vi "Begin.vi"(8 "error in":errorcluster) -> (0 "error out":errorcluster)   [LabVIEW 2016]
doc: "Called before other user functions, this VI is expected to open initial I/O refnums, load in file data, and do all program initialization. Notice that the <B>error out</B> terminal is simply used for data flow. Wiring it to other structures or subVIs ensures that this VI runs first."
uses:
  Robot Global Data.vi
  <vilib>/Rock Robotics/WPI/DriverStation/WPI_DriverStationRobotMode2.ctl
  <vilib>/Rock Robotics/WPI/Joystick/WPI_JoystickDeviceEnum.ctl
  <vilib>/Rock Robotics/Network Tables/NT Write String Array.vi
  <vilib>/Rock Robotics/WPI/SafetyOutput/WPI_SafetyOutputConfigMenu.ctl
  <vilib>/Rock Robotics/WPI/Solenoid/WPI_SolenoidOpenDouble.vi
  <vilib>/Rock Robotics/WPI/RobotDrive/WPI_RobotDriveOpen4MotorWithExistingMotors.vi
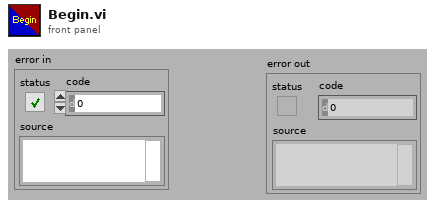
[diagram p1: front panel]
types:
  T1 = typedef "WPI_JoystickDeviceEnum.ctl" = enum16{"USB 0", "USB 1", "USB 2", "USB 3", "USB 4", "USB 5"}
  T2 = typedef "WPI_SafetyOutputConfigMenu.ctl" = enum16{"Enable", "Disable"}
  T3 = typedef "WPI_DriverStationRobotMode2.ctl" = enum16{"Autonomous Disabled", "Autonomous Enabled", "Teleop Disabled", "Teleop Enabled", "Disconnected", "Finish", "Test Disabled", "Test Enabled", "Emergency Stopped"}
  T4 = typedef "WPI_MotorControlDeviceRef.ctl" = cluster{"DeviceStatus":errorcluster, "Type":T5, "PWM":cluster{"PWM Channel":T6, "DeadBand":T7}, "CAN":cluster{"Device Number":u8, "SetOutput VI Ref":variant, "GetOutput VI Ref":variant, "Enable VI Ref":variant, "Disable VI Ref":variant, "Data":variant}, "Invert":bool}
  T5 = typedef "WPI_MotorControlType.ctl" = enum16{"PWM", "CAN"}
  T6 = typedef "FPGA_DIOPWMChannel.ctl" = enum8{"PWM 0", "PWM 1", "PWM 2", "PWM 3", "PWM 4", "PWM 5", "PWM 6", "PWM 7", "PWM 8", "PWM 9", "PWM MXP 0", "PWM MXP 1", "PWM MXP 2", "PWM MXP 3", "PWM MXP 4", "PWM MXP 5", "PWM MXP 6", "PWM MXP 7", "PWM MXP 8", "PWM MXP 9", "Invalid"}
  T7 = typedef "WPI_PWMDeadband.ctl" = cluster{"Name":string, "maxPositivePwm":i32, "minPositivePwm":i32, "centerPwm":i32, "maxNegativePwm":i32, "minNegativePwm":i32, "angularRange":u16}
  T8 = typedef "WPI_JoystickDevRef.ctl" = cluster{"Device":T1}
  T9 = typedef "WPI_RobotDriveDevRef.ctl" = cluster{"DevStatus":errorcluster, "Motors[]":T4[], "Square Inputs":bool, "Max Output":dbl}
  T10 = typedef "WPI_SolenoidDevRef.ctl" = cluster{"DevStatus":errorcluster, "Pneumatics Control Module":u8, "Forward Solenoid Channel":T11, "Reverse Solenoid Channel":T11}
  T11 = typedef "WPI_SolenoidChannel.ctl" = enum8{"Solenoid 0", "Solenoid 1", "Solenoid 2", "Solenoid 3", "Solenoid 4", "Solenoid 5", "Solenoid 6", "Solenoid 7", "Invalid"}
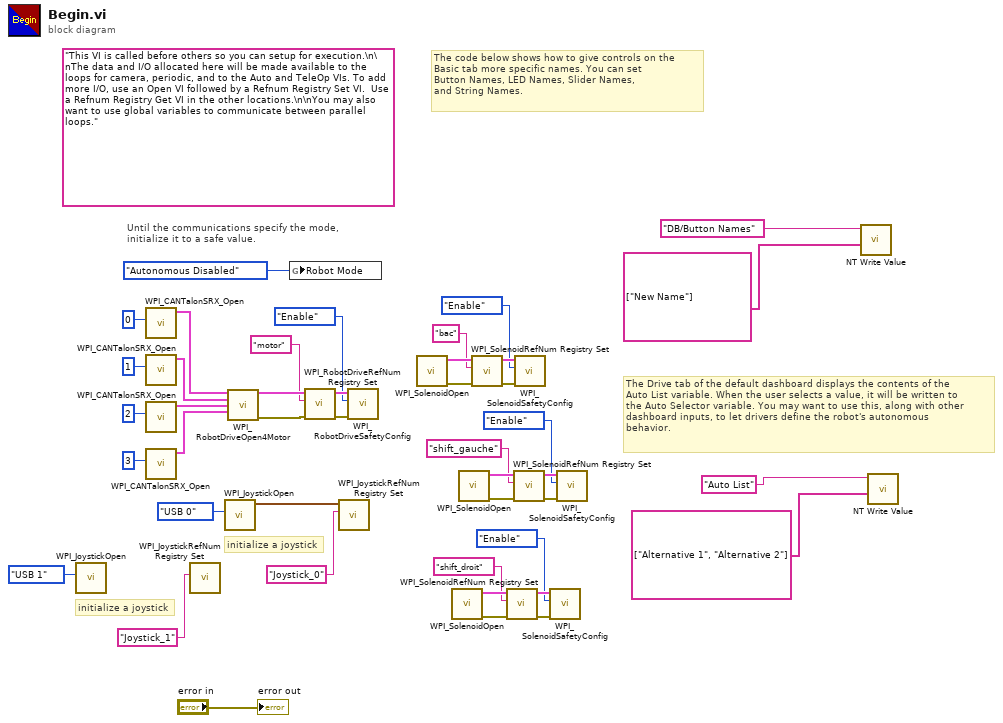
[diagram p0: block diagram]
diagram:
  (unwired) "This VI is called before others so you can setup for execution.\n\nThe data and I/O allocated here will be made available to the loops for camera, periodic, and to the Auto and TeleOp VIs. To add more I/O, use an Open VI followed by a Refnum Registry Set VI.  Use a Refnum Registry Get VI in the other locations.\n\nYou may also want to use global variables to communicate between parallel loops."
  # "initialize a joystick"
  # "The Drive tab of the default dashboard displays the contents of the\nAuto List variable. When the user selects a value, it will be written to\nthe Auto Selector variable. You may want to use this, along with other\ndashboard inputs, to let drivers define the robot's autonomous\nbehavior."
  # "The code below shows how to give controls on the\nBasic tab more specific names. You can set\nButton Names, LED Names, Slider Names,\nand String Names."
  # "initialize a joystick"
  # "Until the communications specify the mode,\ninitialize it to a safe value."
  n1 = call <vilib>:"WPI_JoystickOpen.vi"("JoystickDevice"=WPI_JoystickDeviceEnum."USB 1") -> ()  [unwired: 10 in, 1 out]
  n2 = call <vilib>:"WPI_CANTalonSRX_Open.vi"("Device Number"=u8 0) -> ("CAN Talon SRX Ref"=w29:T4)  [unwired: 9 in, 1 out]
  n3 = call <vilib>:"WPI_CANTalonSRX_Open.vi"("Device Number"=u8 1) -> ("CAN Talon SRX Ref"=w28:T4)  [unwired: 9 in, 1 out]
  n4 = call <vilib>:"WPI_CANTalonSRX_Open.vi"("Device Number"=u8 2) -> ("CAN Talon SRX Ref"=w27:T4)  [unwired: 9 in, 1 out]
  n5 = call <vilib>:"WPI_CANTalonSRX_Open.vi"("Device Number"=u8 3) -> ("CAN Talon SRX Ref"=w26:T4)  [unwired: 9 in, 1 out]
  n6 = call <vilib>:"WPI_JoystickRefNum Registry Set.vi"("refnum name"="Joystick_1") -> ()  [unwired: 9 in, 2 out]
  n7 = call <vilib>:"WPI_JoystickOpen.vi"("JoystickDevice"=WPI_JoystickDeviceEnum."USB 0") -> ("JoystickDevRef"=w42:T8)  [unwired: 10 in]
  n8 = call-poly <vilib>:"WPI_RobotDriveOpen4Motor.vi"("Rear Left Motor Dev Ref"=w29, "Rear Right Motor Dev Ref"=w28, "Front Left Motor Dev Ref"=w27, "Front Right Motor Dev Ref"=w26) -> ("RobotDriveDevRef"=w35:T9, "error out"=w34:errorcluster)  [unwired: 10 in]
  n9 = global write "Robot Global Data.vi" "Robot Mode"(WPI_DriverStationRobotMode2."Autonomous Disabled" ("Robot Mode")) -> ()
  n10 = call <vilib>:"WPI_RobotDriveRefNum Registry Set.vi"("error in (no error)"=w34, "refnum name"="motor", "RobotDriveDevRef"=w35) -> ("error out"=w31:errorcluster, "RobotDriveDevRef"=w32:T9)  [unwired: 7 in]
  n11 = call <vilib>:"WPI_JoystickRefNum Registry Set.vi"("refnum name"="Joystick_0", "JoystickDevRef"=w42) -> ()  [unwired: 8 in, 2 out]
  n12 = call <vilib>:"WPI_RobotDriveSafetyConfig.vi"("error in (no error)"=w31, "mode"=WPI_SafetyOutputConfigMenu."Enable", "RobotDriveDevRef"=w32) -> ()  [unwired: 7 in, 2 out]
  n13 = call-poly <vilib>:"WPI_SolenoidOpen.vi"() -> ("error out"=w20:errorcluster, "SolenoidDevRef"=w21:T10)  [unwired: 10 in]
  n14 = call-poly <vilib>:"WPI_SolenoidOpen.vi"() -> ("error out"=w14:errorcluster, "SolenoidDevRef"=w15:T10)  [unwired: 10 in]
  n15 = call-poly <vilib>:"WPI_SolenoidOpen.vi"() -> ("error out"=w17:errorcluster, "SolenoidDevRef"=w18:T10)  [unwired: 10 in]
  n16 = call <vilib>:"WPI_SolenoidRefNum Registry Set.vi"("error in (no error)"=w20, "refnum name"="bac", "SolenoidDevRef"=w21) -> ("error out"=w12:errorcluster, "SolenoidDevRef"=w11:T10)  [unwired: 7 in]
  n17 = call <vilib>:"WPI_SolenoidRefNum Registry Set.vi"("error in (no error)"=w14, "refnum name"="shift_droit", "SolenoidDevRef"=w15) -> ("error out"=w8:errorcluster, "SolenoidDevRef"=w7:T10)  [unwired: 7 in]
  n18 = call <vilib>:"WPI_SolenoidRefNum Registry Set.vi"("error in (no error)"=w17, "refnum name"="shift_gauche", "SolenoidDevRef"=w18) -> ("error out"=w10:errorcluster, "SolenoidDevRef"=w9:T10)  [unwired: 7 in]
  n19 = call <vilib>:"WPI_SolenoidSafetyConfig.vi"("error in (no error)"=w12, "mode"=WPI_SafetyOutputConfigMenu."Enable", "SolenoidDevRef"=w11) -> ()  [unwired: 7 in, 2 out]
  n20 = call <vilib>:"WPI_SolenoidSafetyConfig.vi"("error in (no error)"=w8, "mode"=WPI_SafetyOutputConfigMenu."Enable", "SolenoidDevRef"=w7) -> ()  [unwired: 7 in, 2 out]
  n21 = call <vilib>:"WPI_SolenoidSafetyConfig.vi"("error in (no error)"=w10, "mode"=WPI_SafetyOutputConfigMenu."Enable", "SolenoidDevRef"=w9) -> ()  [unwired: 7 in, 2 out]
  n22 = call-poly <vilib>:"NT Write Value.vi"("String Array"=string[] ["New Name"], "Name"="DB/Button Names") -> ()  [unwired: 9 in, 1 out]
  n23 = call-poly <vilib>:"NT Write Value.vi"("String Array"=string[] ["Alternative 1", "Alternative 2"], "Name"="Auto List") -> ()  [unwired: 9 in, 1 out]
  "error out" <- "error in"
